vi "proj_czyszczenie_wszystkiego.vi"(6 "Table control 4":refnum<vi>, 7 "Reset":bool, 9 "Table control 3":refnum<vi>, 10 "Table control 2":refnum<vi>, 11 "Table control 1":refnum<vi>) -> (3 "Boolean":bool)   [LabVIEW 2020]
uses:
  <vilib>/Utility/miscctls.llb/LVRowAndColumnTypeDef.ctl
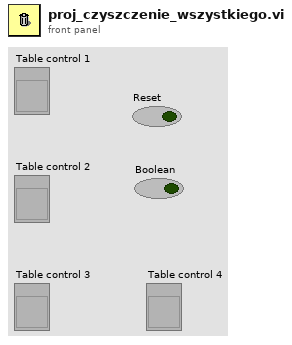
[diagram p1: front panel]
types:
  T1 = typedef "LVRowAndColumnTypeDef.ctl" = cluster{"Row":i32, "Column":i32}
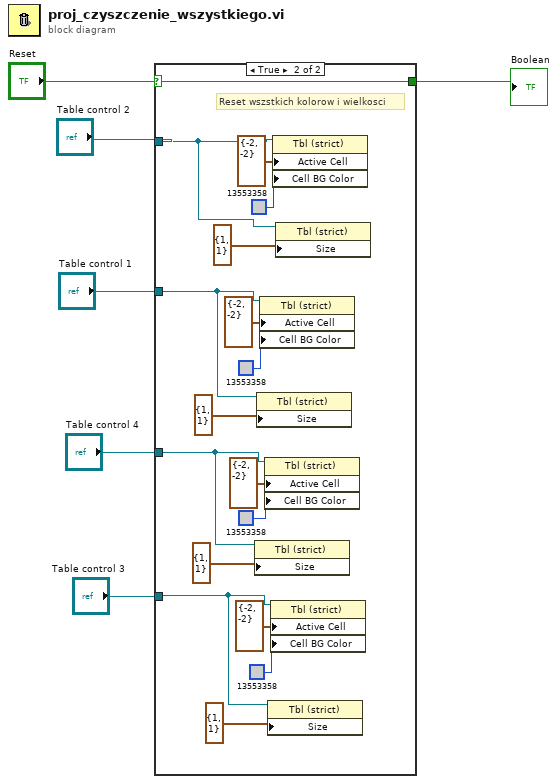
[diagram p0: block diagram]
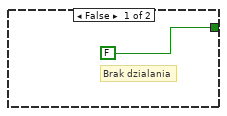
[diagram p2: hidden frame]
diagram:
  n1 = case shown="True" "Reset" {
    selector: "Reset" -> [_ w22]
    tunnel: [FALSE w22] -> w6
    tunnel: "Table control 1" -> [_ w12]
    tunnel: "Table control 2" -> [_ w14]
    tunnel: "Table control 3" -> [_ w8]
    tunnel: "Table control 4" -> [_ w10]
    frame False {
      # "Brak dzialania"
    }
    frame True {
      # "Reset wszstkich kolorow i wielkosci"
      n2 = property on="Property Node" class="Tbl (strict)"(reference=w10, "Size"=cluster{"Row":i32, "Column":i32} {"Row"=1, "Column"=1} ("Edit Position")) -> ()  [unwired: 1 in, 2 out]
      n3 = property on="Property Node" class="Tbl (strict)"(reference=w12, "Size"=cluster{"Row":i32, "Column":i32} {"Row"=1, "Column"=1} ("Edit Position")) -> ()  [unwired: 1 in, 2 out]
      n4 = property on="Property Node" class="Tbl (strict)"(reference=w12, "Active Cell"=T1 {"Row"=-2, "Column"=-2} ("Active Cell:Active Cell"), "Cell BG Color"=u32 13553358 ("Active Cell:Cell Background Color")) -> ()  [unwired: 1 in, 2 out]
      n5 = property on="Property Node" class="Tbl (strict)"(reference=w10, "Active Cell"=T1 {"Row"=-2, "Column"=-2} ("Active Cell:Active Cell"), "Cell BG Color"=u32 13553358 ("Active Cell:Cell Background Color")) -> ()  [unwired: 1 in, 2 out]
      n6 = property on="Property Node" class="Tbl (strict)"(reference=w8, "Size"=cluster{"Row":i32, "Column":i32} {"Row"=1, "Column"=1} ("Edit Position")) -> ()  [unwired: 1 in, 2 out]
      n7 = property on="Property Node" class="Tbl (strict)"(reference=w8, "Active Cell"=T1 {"Row"=-2, "Column"=-2} ("Active Cell:Active Cell"), "Cell BG Color"=u32 13553358 ("Active Cell:Cell Background Color")) -> ()  [unwired: 1 in, 2 out]
      n8 = property on="Property Node" class="Tbl (strict)"(reference=w14, "Active Cell"=T1 {"Row"=-2, "Column"=-2} ("Active Cell:Active Cell"), "Cell BG Color"=u32 13553358 ("Active Cell:Cell Background Color")) -> ()  [unwired: 1 in, 2 out]
      n9 = property on="Property Node" class="Tbl (strict)"(reference=w14, "Size"=cluster{"Row":i32, "Column":i32} {"Row"=1, "Column"=1} ("Edit Position")) -> ()  [unwired: 1 in, 2 out]
    }
  }
  "Boolean" <- w6
